vi "HP81110A Set Display.vi"(8 "error in (no error)":errorcluster, 10 "Display (F:Off)":bool, 11 "VISA session":refnum<visa-resource-name>) -> (0 "error out":errorcluster, 3 "dup VISA session":refnum<visa-resource-name>)   [LabVIEW 2015]
doc: "This VI turns the frontpanel display on and off. Switching off the display improves the programming speed of the instrument."
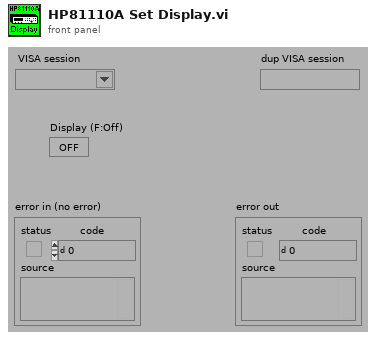
[diagram p1: front panel]
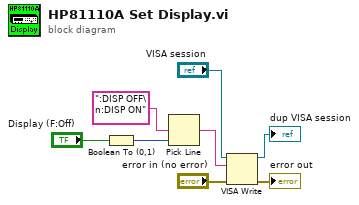
[diagram p0: block diagram]
diagram:
  n1 = Boolean To (0,1)(Boolean="Display (F:Off)") -> (0, 1=w2:i16)
  n2 = Pick Line(multi-line string=":DISP OFF\n:DISP ON", line index=w2) -> (output string=w5:string)  [unwired: 1 out]
  n3 = VISA Write(VISA resource name="VISA session", write buffer=w5, error in (no error)="error in (no error)") -> (VISA resource name out=→"dup VISA session":refnum<visa-resource-name>, error out=→"error out":errorcluster)  [unwired: 1 out]
